vi "export results.vi"(9 "Graph array":cluster{"output":dbl[], "output":dbl[]}[](array[cluster])=[{"output"=array[1831 elements], "output"=array[1831 elements]}, {"output"=array[1238 elements], "output"=array[1238 elements]}, {"output"=array[1485 elements], "output"=array[1485 elements]}], 10 "Y-columns":dbl[](array[numeric])=[9.0], 11 "selected files2":T1(array[cluster])=[{"String"="Cell9_SS,,.003.txt", "Boolean"=TRUE, "begin"=0, "length"=1831, "Numeric"=1.0}, {"String"="Cell9_SS,,.004.txt", "Boolean"=TRUE, "begin"=0, "length"=1238, "Numeric"=1.0}, {"String"="Cell9_SS,,.005.txt", "Boolean"=TRUE, "begin"=0, "length"=1485, "Numeric"=1.0}]) -> ()   [LabVIEW 2020]
panel:
  out "Data summary":string="There are 3 datasets with 1 columns (y-axis) for each.\n\nProvide  (1) x-axis title (2) column names common for each dataset. If lempty, default names will be used.\n\nEach dataset can be either numbered as shown in the graph or labeled."
  in  "(6) Done":bool
  in  "(3) use custom \nvariables?":bool
  in  "(4) variables\n (should be filled)":string
  in  "file path (dialog if empty)":path
  in  "window name (no special character)":string="Data1"
  in  "(5) export method":T2(ring)=enum."Save to Igor ITX"
  in  "(2) Y-column names":string[](array[string])=["mr"]
  in  "(1) x-axis title":string="field"
  out "new file path (Not A Path if cancelled) 2":path=path "C:/work/data/Magnet runs/Cell 9 2017 Summer School/test_window2.itx"
  # "(for Origin or Igor files)"
  # "(each column names should be filled for Igor ITX files)"
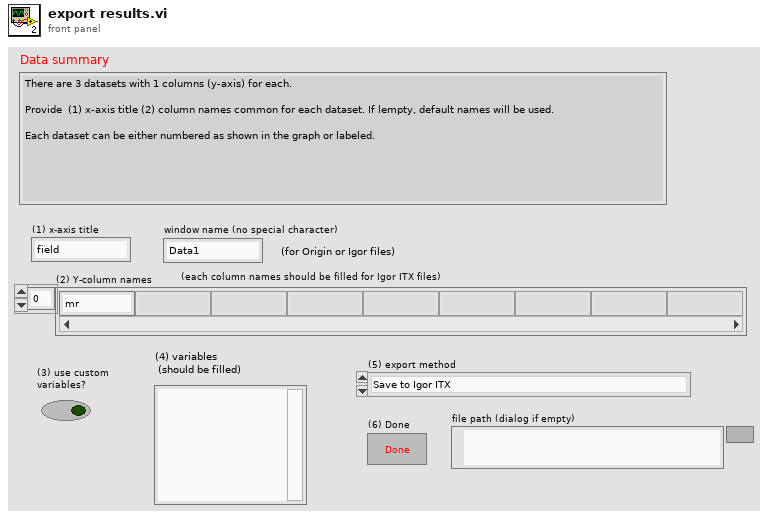
[diagram p1: front panel]
types:
  T1 = cluster{"String":string, "Boolean":bool, "begin":u32, "length":u32, "Numeric":dbl}[]
  T2 = enum16{"do not export", "Save to Igor ITX", "Save as Ascill file", "write to clipboard"}
  T3 = enum16{"Save as Ascill file", "write to clipboard", "do not export"}
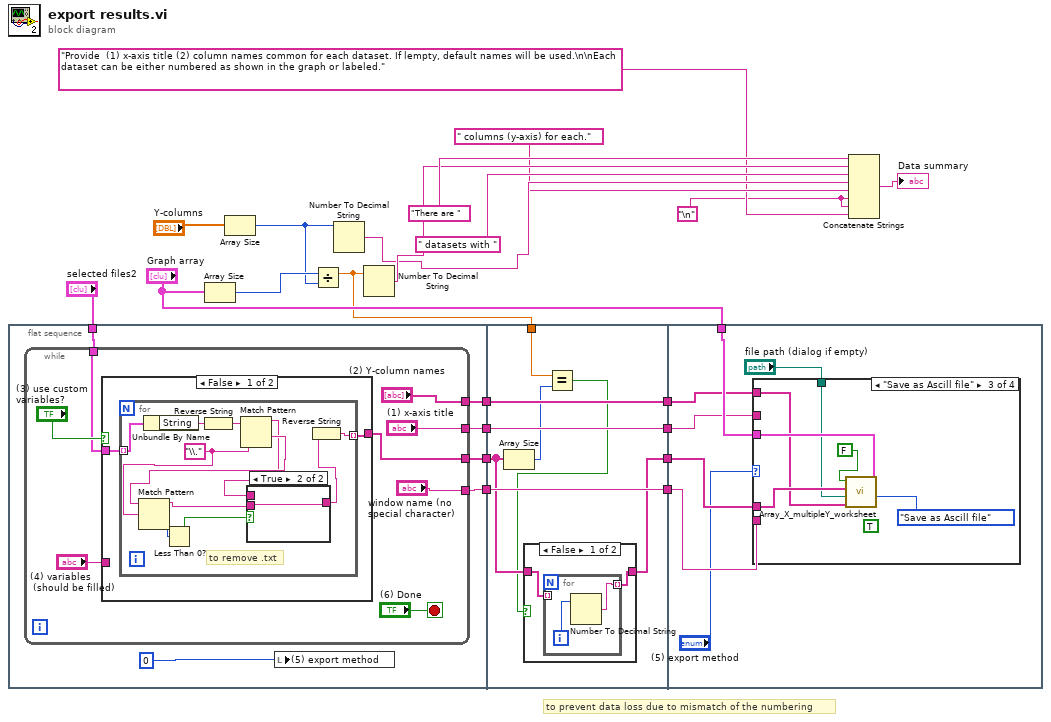
[diagram p0: block diagram]
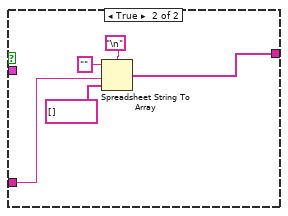
[diagram p3: hidden frame]
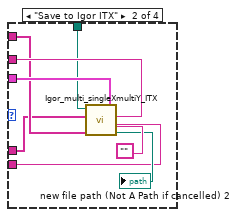
[diagram p6: hidden frame]
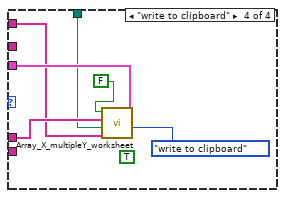
[diagram p7: hidden frame]
diagram:
  w10 = "\n"
  # "to prevent data loss due to mismatch of the numbering"
  n1 = flat-sequence {
    tunnel: [w28] -> w9
    tunnel: [w27] -> w7
    tunnel: [w26] -> w5
    tunnel: [w25] -> w3
    tunnel: "selected files2" -> [w24]
    tunnel: w9 -> [w64]
    tunnel: [w64] -> w8
    tunnel: w7 -> [w63]
    tunnel: [w63] -> w6
    tunnel: w5 -> [w62]
    tunnel: [w62] -> w4
    tunnel: w3 -> [w59]
    tunnel: w2 -> [w60]
    tunnel: [w58] -> w1
    tunnel: "Graph array" -> [w76]
    tunnel: w8 -> [w75]
    tunnel: w6 -> [w74]
    tunnel: w4 -> [w73]
    tunnel: w1 -> [w72]
    frame #0 {
      n2 = while {
        tunnel: ["(2) Y-column names"] -> w28
        tunnel: ["(1) x-axis title"] -> w27
        tunnel: ["window name (no special character)"] -> w26
        tunnel: [w32] -> w25
        tunnel: w24 -> [w30]
        stop <- "(6) Done" stop-if-true
        n3 = case shown="False" "(3) use custom \nvariables?" {
          tunnel: [w38 w53] -> w32
          tunnel: w30 -> [w37 _]
          tunnel: "(4) variables\n (should be filled)" -> [_ w52]
          frame False {
            n4 = for {
              tunnel: [w47] -> w38 mode=indexing
              tunnel: w37 -> [w46] mode=indexing
              w45 = "\\." ("regular expression")
              # "to remove .txt"
              n5 = Unbundle By Name(w46) -> ("String"=w49:string)
              n6 = Reverse String(1:w49) -> (0:w48:string)
              n7 = Match Pattern(string=w48, regular expression=w45) -> (before substring=w39:string, after substring=w40:string)  [unwired: 1 in, 2 out]
              n8 = Match Pattern(string=w40, regular expression=w45) -> (before substring=w41:string, offset past match=w43:i32)  [unwired: 1 in, 2 out]
              n9 = Less Than 0?(x=w43) -> (x < 0?=w42:bool)
              n10 = case shown="True" w42 {
                tunnel: w39 -> [_ w51]
                tunnel: [w50 w51] -> w44
                tunnel: w41 -> [w50 _]
                frame False {
                }
                frame True {
                }
              }
              n11 = Reverse String(1:w44) -> (0:w47:string)
            }
          }
          frame True {
            n12 = Spreadsheet String To Array(delimiter (Tab)="\n", format string="", spreadsheet string=w52, array type (2D Dbl)=string[] []) -> (array=w53:string[])
          }
        }
      }
      n13 = local write "(5) export method"(0) -> ()
    }
    frame #1 {
      n14 = Array Size(array=w59) -> (size(s)=w61:i32)
      n15 = Equal?(x=w60, y=w61) -> (x = y?=w57:bool)
      n16 = case shown="False" w57 {
        tunnel: w59 -> [w66 w69]
        tunnel: [w65 w69] -> w58
        frame False {
          n17 = for {
            tunnel: w66 -> [_] mode=indexing
            tunnel: [w67] -> w65 mode=indexing
            i -> [w68]
            n18 = Number To Decimal String(number=w68) -> (decimal integer string=w67:string)  [unwired: 1 in]
          }
        }
        frame True {
        }
      }
    }
    frame #2 {
      n19 = case shown="\"Save as Ascill file\"" "(5) export method" {
        tunnel: w76 -> [_ w81 w89 w95]
        tunnel: "file path (dialog if empty)" -> [_ w80 w87 w93]
        tunnel: w75 -> [_ w78 w86 w92]
        tunnel: w74 -> [_ w82 _ _]
        tunnel: w73 -> [_ w79 _ _]
        tunnel: w72 -> [_ w77 w88 w94]
        frame "do not export", Default {
        }
        frame "Save to Igor ITX" {
          n20 = call "Igor_multi_singleXmultiY_ITX.vi"("message"="", "x-column name"=w82, "graph file"=w81, "Y-column names"=w78, "window name"=w79, "column extension"=w77, "file"=w80) -> ("new file path (Not A Path if cancelled)"=→"new file path (Not A Path if cancelled) 2":path)
        }
        frame "Save as Ascill file" {
          (unwired) TRUE ("save ascii")
          n21 = call "Array_X_multipleY_worksheet.vi"("Sort?"=FALSE, "column extension"=w88, "file path (dialog if empty)"=w87, "Y-column names"=w86, "graph file"=w89, "export"=T3."Save as Ascill file") -> ()  [unwired: 1 in, 2 out]
        }
        frame "write to clipboard" {
          (unwired) TRUE ("save ascii")
          n22 = call "Array_X_multipleY_worksheet.vi"("Sort?"=FALSE, "column extension"=w94, "file path (dialog if empty)"=w93, "Y-column names"=w92, "graph file"=w95, "export"=T3."write to clipboard") -> ()  [unwired: 1 in, 2 out]
        }
      }
    }
  }
  n23 = Array Size(array="Graph array") -> (size(s)=w19:i32)
  n24 = Array Size(array="Y-columns") -> (size(s)=w15:i32)
  n25 = Divide(x=w19, y=w15) -> (x/y=w2:dbl)
  n26 = Number To Decimal String(number=w15) -> (decimal integer string=w14:string)  [unwired: 1 in]
  n27 = Number To Decimal String(number=w2) -> (decimal integer string=w17:string)  [unwired: 1 in]
  n28 = Concatenate Strings("There are ", w17, " datasets with " ("string"), w14, " columns (y-axis) for each." ("string"), w10, w10, "Provide  (1) x-axis title (2) column names common for each dataset. If lempty, default names will be used.\n\nEach dataset can be either numbered as shown in the graph or labeled." ("string")) -> (→"Data summary":string)
